vi "hmi3.vi"() -> ()   [LabVIEW 2017]
doc: "Demonstrates how to write and receive CAN frames via the Network Interface on the same port. \n\nTo write and receive frames via the Network Interface:\n- select the CAN Network Interface (i.e. CAN0, CAN1, etc.)\n- select the Baud Rate\n- run the VI\n- press the write button to write frames to the can bus\n\nEnable RTR Button to send a Remote Transmission Request or to simply send an empty Frame to request an Answer Frame from a connected device.\n\nEnable Extended Button to write extended Identifier Format. This is done by setting the 30th bit to enable extended format with the driver."
uses:
  <vilib>/nican/nican.llb/CanFrameTimed.ctl
  <vilib>/nican/nican.llb/ncNetAttr.ctl
panel:
  in  "binFile":path=path "C:/Users/twalling/Desktop/hubert-master/hubert-master/examples/02-blinky/Debug/blinky.bin"
  out "msgDataDl":T1[](array[typedef]) {"Data" format="%.0x"; "ArbitrationId" format="%.0x"; "Timestamp" format="%<%I:%M:%S%3u %p\n%m/%d/%Y>T"}
  in  "Program":bool
  in  "InitForceUpdate?":bool
  in  "IND2":bool
  in  "IND1":bool
  out "Data":u8[](array[numeric])
  out "Heartbeat":u16 format="%04x"
  in  "interface":string(combo)="CAN0" caption="Interface"
  in  "shutdown":bool
  # "PRESS AND HOLD"
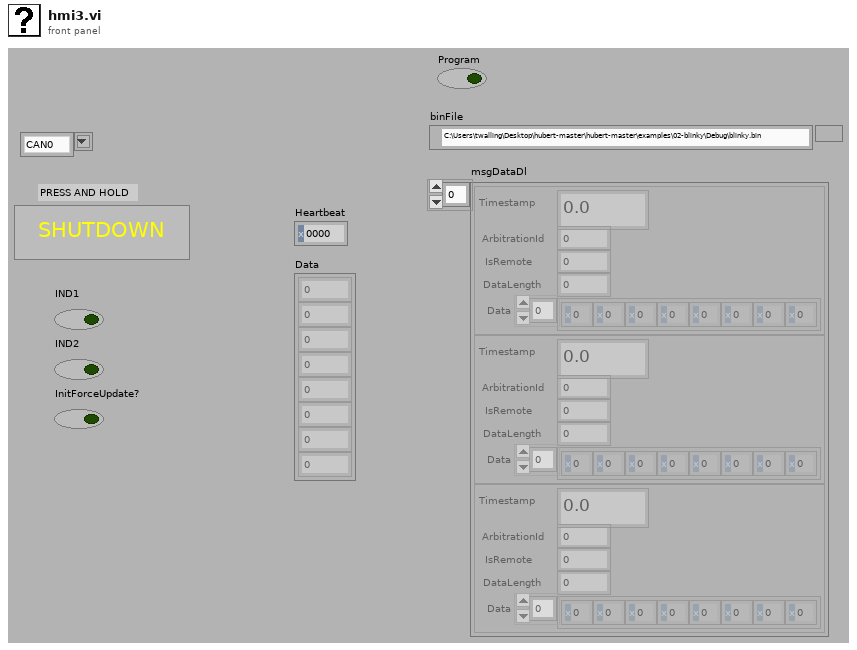
[diagram p1: front panel]
types:
  T1 = typedef "CanFrameTimed.ctl" = cluster{"Timestamp":dbl, "ArbitrationId":u32, "IsRemote":u8, "DataLength":u8, "Data":u8[]}
  T2 = typedef "ncNetAttr.ctl" = cluster{"Start On Open":enum32{"FALSE", "TRUE"}, "Baud Rate":u32, "Read Queue Length":u32, "Write Queue Length":u32, "Standard Comparator":u32, "Standard Mask":u32, "Extended Comparator":u32, "Extended Mask":u32}
  T3 = typedef "xobjhandle.ctl" = u32
  T4 = cluster{dbl, u32, "IsRemote":u8, "DataLength":u8, u8[]}
  T5 = cluster{dbl, u32, "IsRemote":u8, "DataLength":u8, u8[]}[]
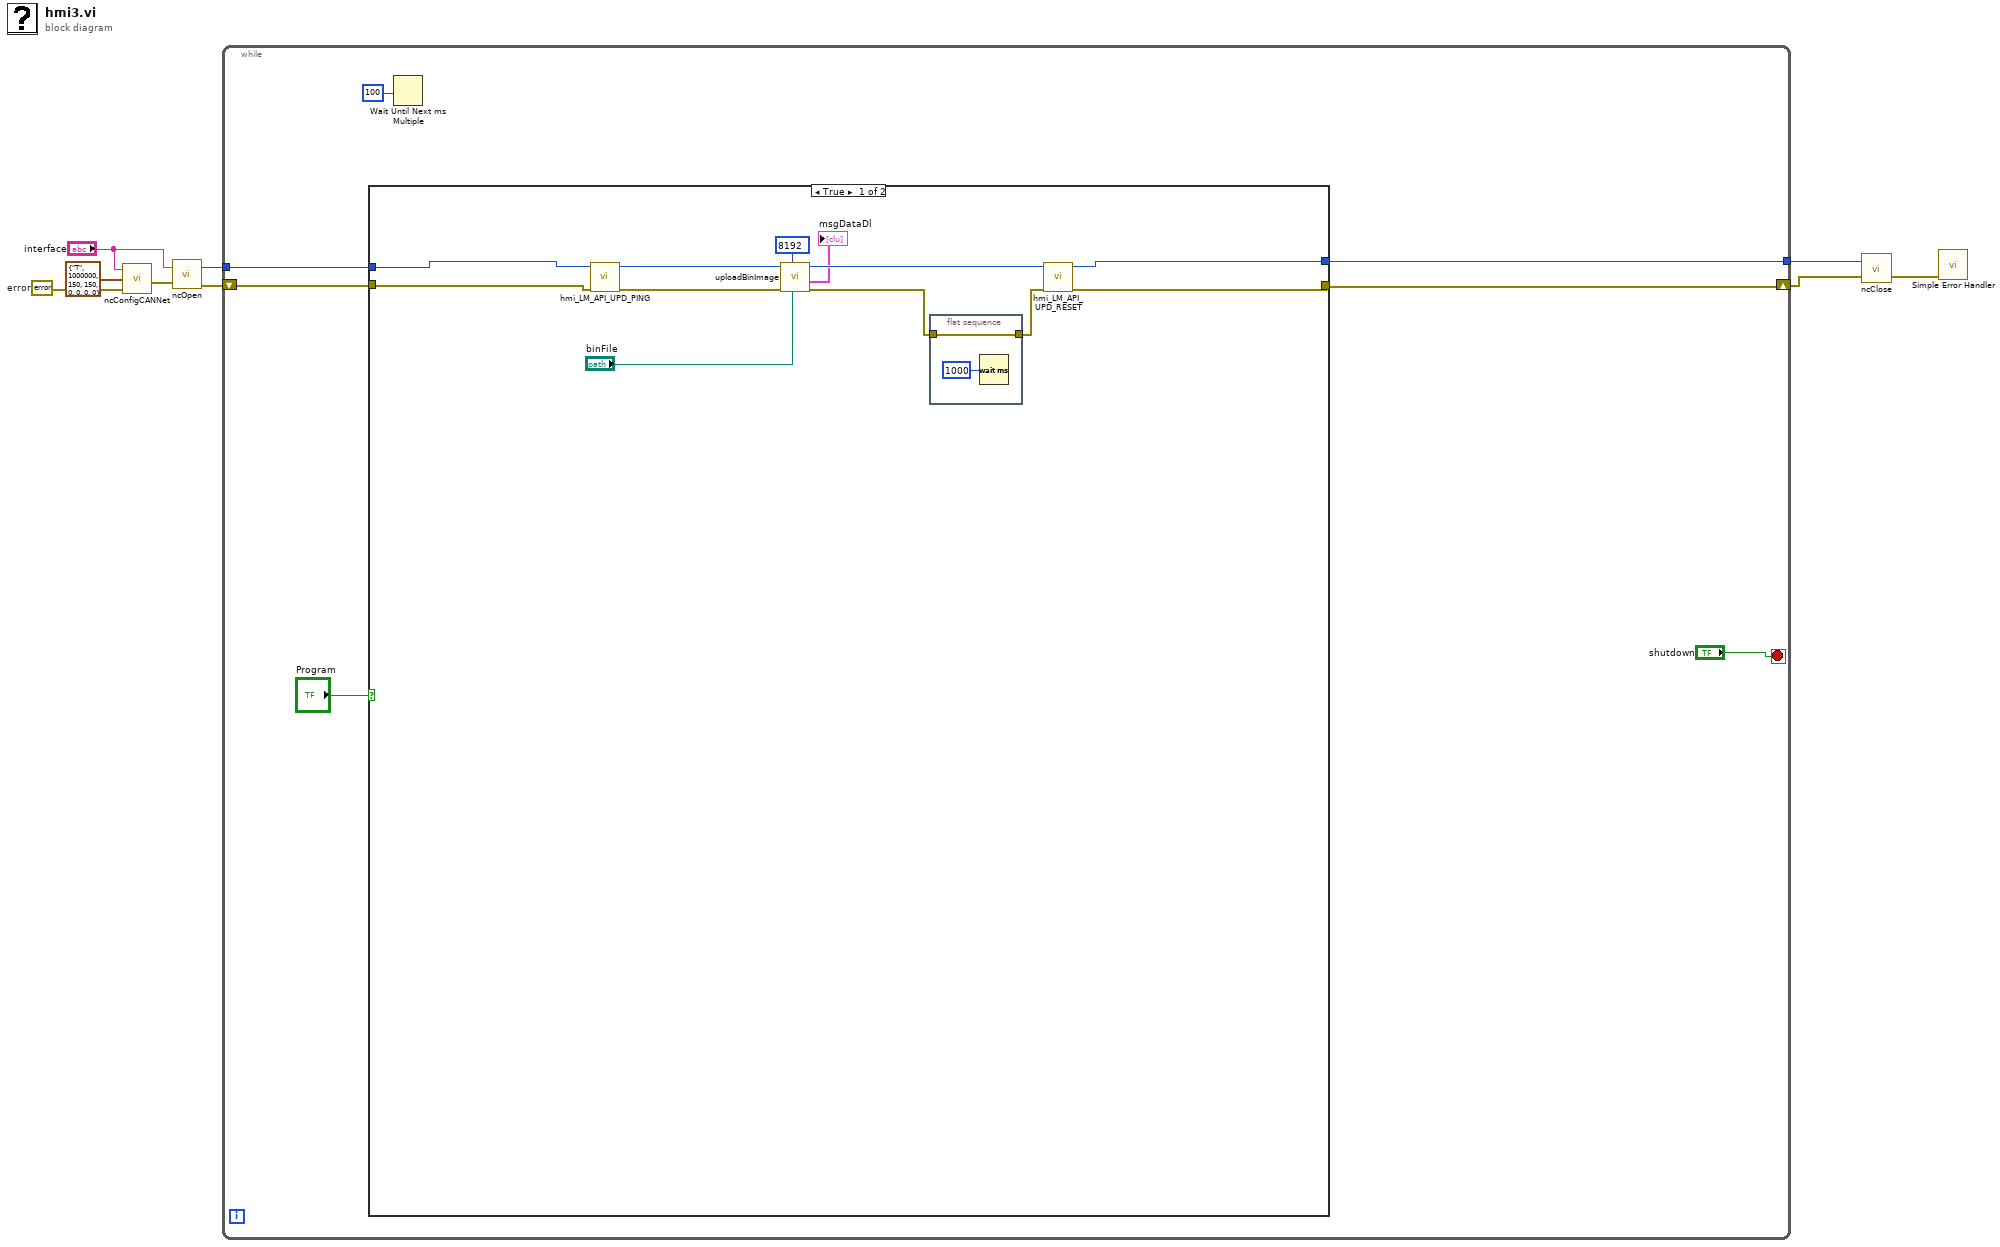
[diagram p0: block diagram]
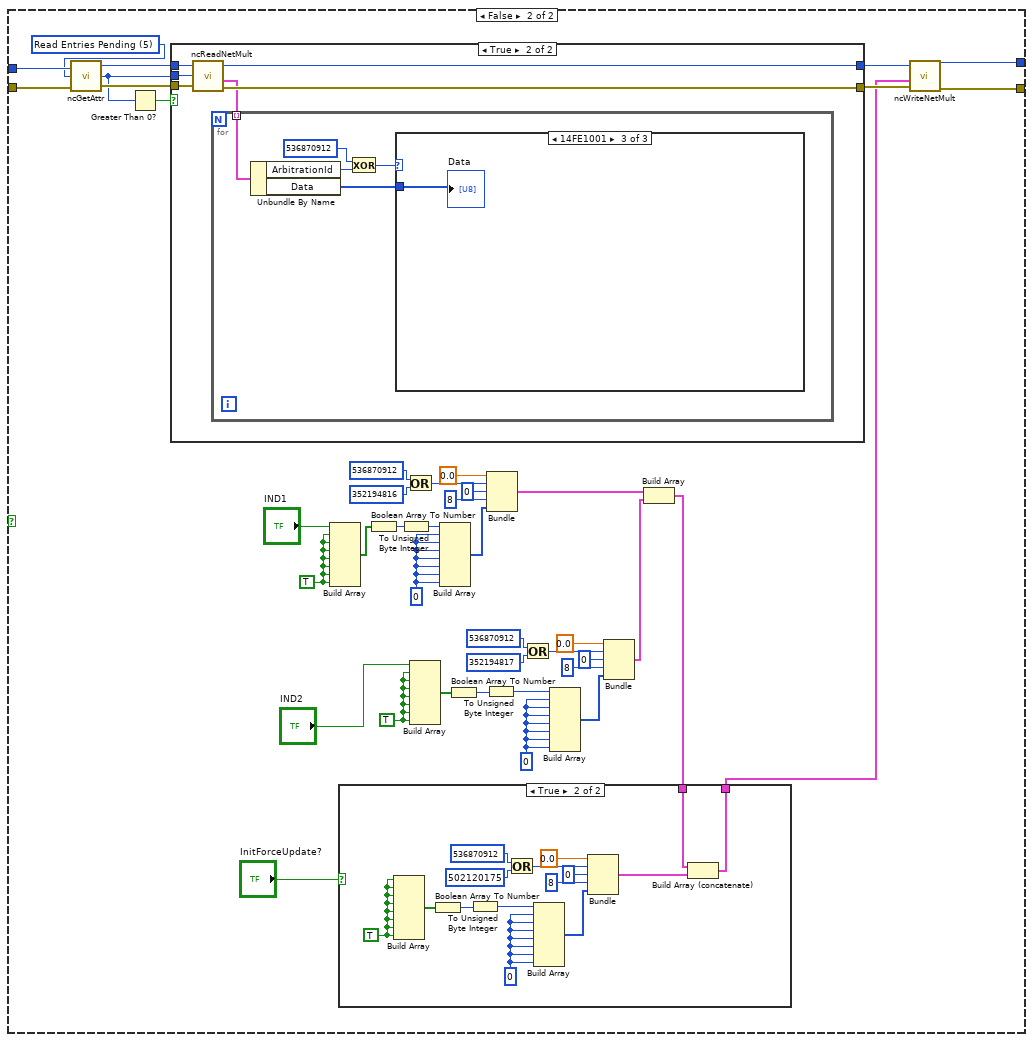
[diagram p2: hidden frame]
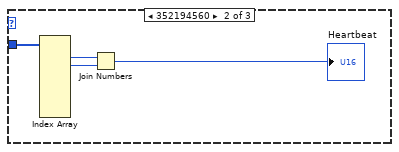
[diagram p6: hidden frame]
diagram:
  w5 = errorcluster {"status"=FALSE, "code"=0, "source"=""}  # error
  n1 = call <vilib>:"ncConfigCANNet.vi"("Error in"=w5, "CAN Network Interface Config"=T2 {"Start On Open"=enum."TRUE", "Baud Rate"=1000000, "Read Queue Length"=150, "Write Queue Length"=150, "Standard Comparator"=0, "Standard Mask"=0, "Extended Comparator"=0, "Extended Mask"=0}, "ObjName"="interface") -> ("Error out"=w6:errorcluster)  [unwired: 2 in]
  n2 = call <vilib>:"ncOpen.vi"("Error in"=w6, "ObjName"="interface") -> ("Error out"=w9:errorcluster, "ObjHandle out"=w7:T3)
  n3 = while {
    tunnel: w7 -> [w14]
    tunnel: [w15] -> w2
    shift-right: [w16] -> w1
    shift-left: w9 -> [w13]
    stop <- "shutdown" stop-if-true
    n4 = case shown="True" "Program" {
      tunnel: [w17 w72] -> w16
      tunnel: [w18 w71] -> w15
      tunnel: w14 -> [w20 w66]
      tunnel: w13 -> [w19 w65]
      frame True {
        n5 = call "hmi_LM_API_UPD_PING.vi"("Error in"=w19, "canSession"=w20) -> ("Error out"=w26:errorcluster, "canSession"=w27:T3)  [unwired: 7 in, 1 out]
        n6 = call "uploadBinImage.vi"("binFile"="binFile", "dloadAddr"=u32 8192 ("dloadSize"), "Error in"=w26, "canSession"=w27) -> ("Error out"=w25:errorcluster, "msgData"=→"msgDataDl":T1[], "canSession"=w24:T3)  [unwired: 5 in]
        n7 = flat-sequence {
          tunnel: w25 -> [w30]
          tunnel: [w30] -> w28
          frame #0 {
            n8 = Wait (ms)(milliseconds to wait=u32 1000) -> ()  [unwired: 1 out]
          }
        }
        n9 = call "hmi_LM_API_UPD_RESET.vi"("Error in"=w28, "canSession"=w24) -> ("Error out"=w17:errorcluster, "canSession"=w18:T3)  [unwired: 8 in]
      }
      frame False {
        w41 = TRUE ("element")
        w43 = TRUE ("element")
        w46 = u8 0
        w54 = u8 0
        w62 = u32 5 items=["(reserved)", "Protocol Version", "Software Version", "Object State", "(reserved)", "Read Entries Pending", "Write Entries Pending", "ReadMult Size for Notification", "Listen Only?", "Self Reception?", "Transmit Error Counter", "Receive Error Counter", "Single Shot Transmit?", "Series 2 Filter Mode", "Series 2 Mask", "Series 2 Comparator", "Serial Number", "Form Factor", "Series", "Transceiver Type", "Interface Number", "Series 2 Error/Arb Capture", "Transceiver Mode", "Transceiver External Outputs", "Transceiver External Inputs", "Start Trigger Behavior", "Log Comm Warnings", "User RTSI Frame", "Transmit Mode", "Log Start Trigger?", "Timestamp Format", "Master Timebase Rate", "Virtual Bus Timing"] ("AttrId")
        n10 = call <vilib>:"ncGetAttr.vi"("Error in"=w65, "AttrId"=w62, "ObjHandle in"=w66) -> ("Error out"=w70:errorcluster, "AttrValue"=w67:u32, "ObjHandle out"=w69:T3)
        n11 = Greater Than 0?(x=w67) -> (x > 0?=w68:bool)
        n12 = case shown="True" w68 {
          tunnel: [w89 w96] -> w63
          tunnel: [w90 w95] -> w64
          tunnel: w67 -> [_ w94]
          tunnel: w70 -> [w89 w93]
          tunnel: w69 -> [w90 w92]
          frame False {
          }
          frame True {
            n13 = call <vilib>:"ncReadNetMult.vi"("ObjHandle in"=w92, "Requested Number of Frames"=w94, "Error in"=w93) -> ("ObjHandle out"=w95:T3, "Data"=w91:T1[], "Error out"=w96:errorcluster)  [unwired: 1 out]
            n14 = for {
              tunnel: w91 -> [w101] mode=indexing
              n15 = Unbundle By Name(w101) -> ("ArbitrationId"=w99:u32, "Data"=w97:u8[])
              n16 = Exclusive Or(1:w99, 2:u32 536870912 ("y")) -> (0:w98:u32)
              n17 = case shown="14FE1001" w98 {
                tunnel: w97 -> [_ w105 w106]
                frame Default {
                }
                frame 352194560 {
                  n18 = Index Array(array=w105) -> (element #1=w103:u8, element #2=w104:u8)  [unwired: 8 in, 6 out]
                  n19 = Join Numbers(hi=w103, lo=w104) -> ((hi.lo)=→"Heartbeat":u16)
                }
                frame 352194561 {
                  "Data" <- w106
                }
              }
            }
          }
        }
        n20 = Build Array("IND1", w43, w43, w43, w43, w43, w43, w43) -> (w37:bool[])
        n21 = Boolean Array To Number(Boolean array=w37) -> (number=w39:u32)
        n22 = To Unsigned Byte Integer(number=w39) -> (unsigned 8bit integer=w38:u8)
        n23 = Or(x=u32 536870912 ("y"), y=u32 352194816) -> (x .or. y?=w52:u32)
        n24 = Build Array("IND2", w41, w41, w41, w41, w41, w41, w41) -> (w42:bool[])
        n25 = Build Array(w38, w46, w46, w46, w46, w46, w46, w46) -> (w48:u8[])
        n26 = Boolean Array To Number(Boolean array=w42) -> (number=w35:u32)
        n27 = To Unsigned Byte Integer(number=w35) -> (unsigned 8bit integer=w36:u8)
        n28 = Bundle(0.0, w52, "IsRemote"=u8 0, "DataLength"=u8 8, w48) -> (w45:T4)  [unwired: 1 in]
        n29 = Or(x=u32 536870912 ("y"), y=u32 352194817) -> (x .or. y?=w60:u32)
        n30 = Build Array(w36, w54, w54, w54, w54, w54, w54, w54) -> (w56:u8[])
        n31 = Bundle(0.0, w60, "IsRemote"=u8 0, "DataLength"=u8 8, w56) -> (w33:T4)  [unwired: 1 in]
        n32 = Build Array(w45, w33) -> (w32:T5)
        n33 = case shown="True" "InitForceUpdate?" {
          tunnel: w32 -> [w73 w77]
          tunnel: [w73 w75] -> w31
          frame False {
          }
          frame True {
            w74 = TRUE ("element")
            w85 = u8 0
            n34 = Build Array(w74, w74, w74, w74, w74, w74, w74, w74) -> (w86:bool[])
            n35 = Boolean Array To Number(Boolean array=w86) -> (number=w88:u32)
            n36 = To Unsigned Byte Integer(number=w88) -> (unsigned 8bit integer=w87:u8)
            n37 = Or(x=u32 536870912 ("y"), y=u32 502120175) -> (x .or. y?=w79:u32)
            n38 = Build Array(w87, w85, w85, w85, w85, w85, w85, w85) -> (w83:u8[])
            n39 = Bundle(0.0, w79, "IsRemote"=u8 0, "DataLength"=u8 8, w83) -> (w76:T4)  [unwired: 1 in]
            n40 = Build Array (concatenate)(w77, w76) -> (w75:T5)
          }
        }
        n41 = call <vilib>:"ncWriteNetMult.vi"("Error in"=w63, "Data"=w31, "ObjHandle in"=w64) -> ("Error out"=w72:errorcluster, "ObjHandle out"=w71:T3)  [unwired: 7 in]
      }
    }
    n42 = Wait Until Next ms Multiple(millisecond multiple=u32 100) -> ()  [unwired: 1 out]
  }
  n43 = call <vilib>:"ncClose.vi"("Error in"=w1, "ObjHandle in"=w2) -> ("Error out"=w3:errorcluster)  [unwired: 1 in]
  n44 = call <vilib>:"Simple Error Handler.vi"("error in (no error)"=w3) -> ()  [unwired: 4 in, 5 out]
